vi "Repopulate Component Lists.vi"(8 "error in (no error)":errorcluster, 11 "MLA in":refnum<class "MLA.lvclass">) -> (0 "error out":errorcluster, 3 "MLA out":refnum<class "MLA.lvclass">)   [LabVIEW 2017]
uses:
  MLA/MLA.lvclass
  Typedefs/Commands.ctl
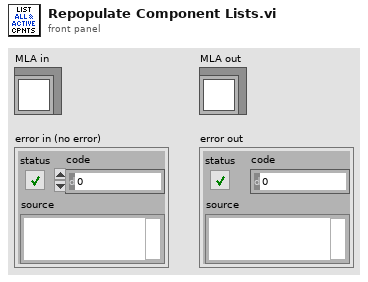
[diagram p1: front panel]
types:
  T1 = typedef "Commands.ctl" = enum16{"refresh", "listActiveComponents", "listComponents", "loadComponent", "unloadComponent", "swapComponent"}
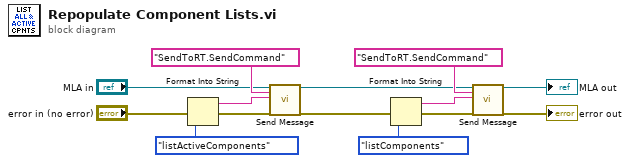
[diagram p0: block diagram]
diagram:
  n1 = Format Into String(error in="error in (no error)", Commands."listActiveComponents") -> (resulting string=w13:string, error out=w14:errorcluster)  [unwired: 2 in]
  n2 = call-dynamic "Send Message.vi"("MLA"="MLA in", "Message"="SendToRT.SendCommand", "Param 1"=w13, "error in (no error)"=w14) -> ("MLA"=w3:refnum<class "MLA.lvclass">, "error out"=w6:errorcluster)  [unwired: 14 in]
  n3 = Format Into String(error in=w6, Commands."listComponents") -> (resulting string=w9:string, error out=w10:errorcluster)  [unwired: 2 in]
  n4 = call-dynamic "Send Message.vi"("MLA"=w3, "Message"="SendToRT.SendCommand", "Param 1"=w9, "error in (no error)"=w10) -> ("MLA"=→"MLA out":refnum<class "MLA.lvclass">, "error out"=→"error out":errorcluster)  [unwired: 14 in]
